vi "Caller.vi"(0 "Arithemetic Operation in":refnum<class "Arithemetic Operation.lvclass">, 2 "DVR":refnum<data-value>, 5 "Sub Panel":refnum<vi>, 7 "State":refnum<user-event>, 9 "Class Data":refnum<user-event>, 11 "Error In":errorcluster) -> (4 "Arithemetic Operation out":refnum<class "Arithemetic Operation.lvclass">, 15 "Error Out":errorcluster)   [LabVIEW 2023, in "Arithemetic Operation.lvclass"]
doc: "The VI is the over riding VI that calls another VI asynchronously."
uses:
  Arithemetic Operation.lvclass
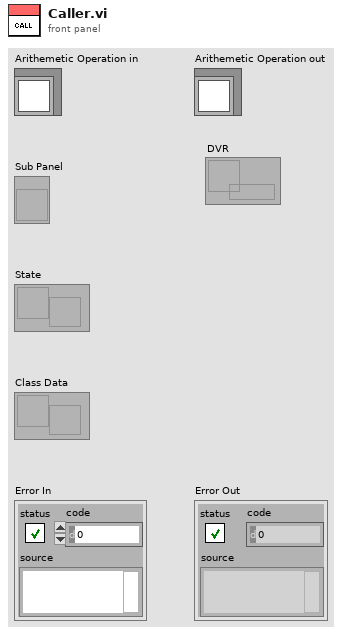
[diagram p1: front panel]
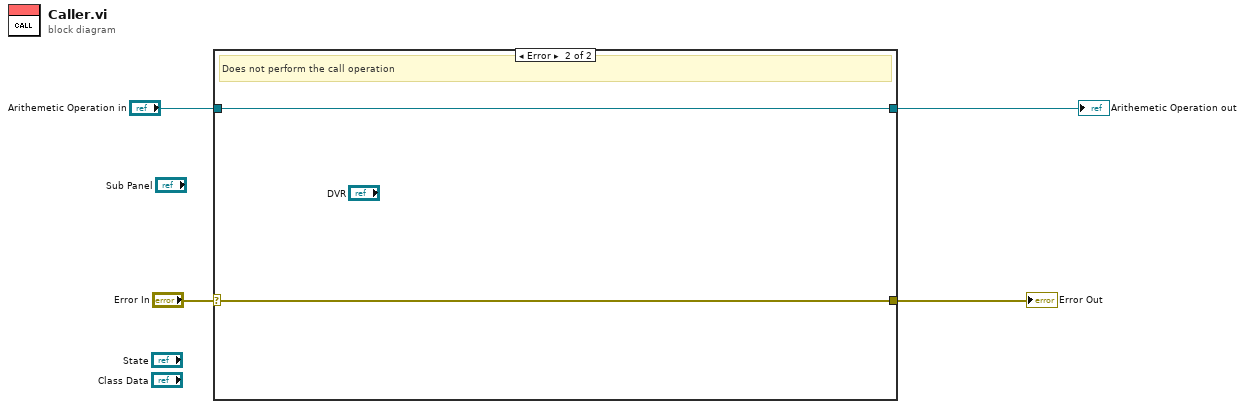
[diagram p0: block diagram]
diagram:
  n1 = case shown="Error" "Error In" {
    selector: "Error In" -> [w6 w8]
    tunnel: [w6 w8] -> w4
    tunnel: [w5 w7] -> w1
    tunnel: "Arithemetic Operation in" -> [w5 w7]
    frame No Error {
      # "Calls the Addition operation UI asynchronously"
    }
    frame Error {
      # "Does not perform the call operation"
    }
  }
  "Error Out" <- w4
  "Arithemetic Operation out" <- w1
